vi "Merge Traces.vi"(8 "error in (no error)":errorcluster, 10 "Historical Data from Logging Database":T1, 11 "Historical Data from Archive Database":T1) -> (0 "error out":errorcluster, 3 "Merged Historical Trace":T1)   [LabVIEW 2024]
doc: "Merges the traces from the logging database and the archive database."
uses:
  Controls/Client/Historical Data.ctl
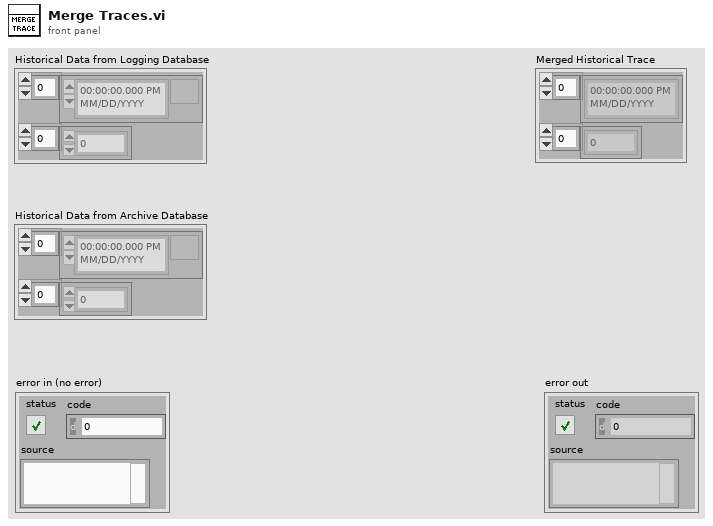
[diagram p1: front panel]
types:
  T1 = typedef "Historical Data.ctl" = cluster{"timestamps":timestamp[], "data":dbl[]}
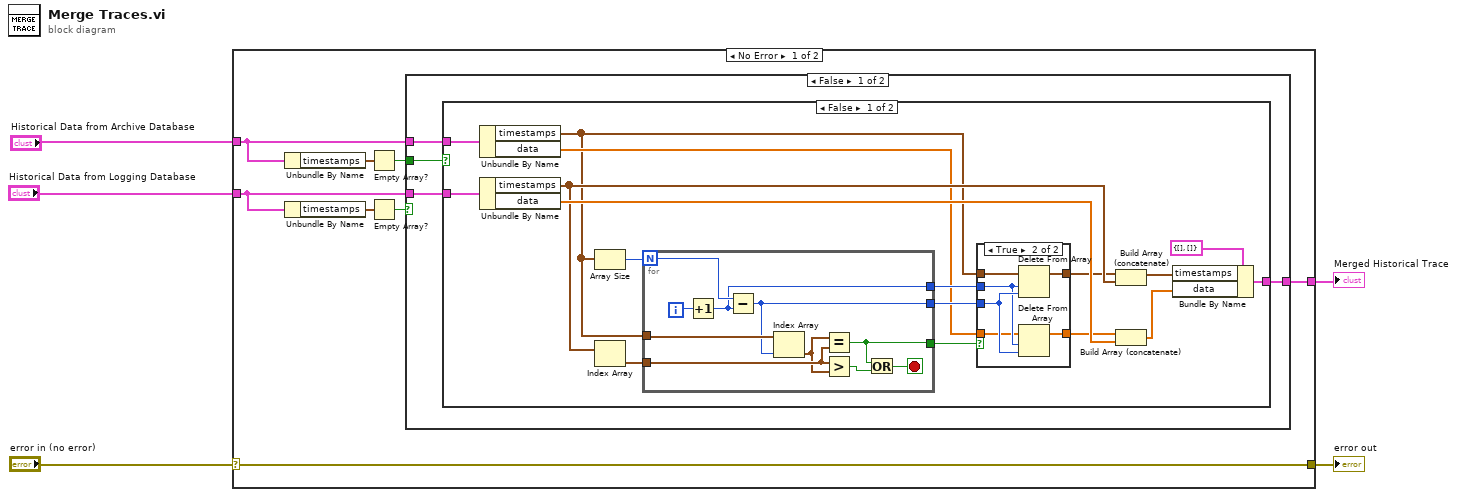
[diagram p0: block diagram]
diagram:
  n1 = case shown="No Error" "error in (no error)" {
    selector: "error in (no error)" -> [w6 w55]
    tunnel: [w6 w55] -> w4
    tunnel: "Historical Data from Archive Database" -> [w9 _]
    tunnel: "Historical Data from Logging Database" -> [w8 _]
    tunnel: [w7 _] -> w1
    frame No Error {
      n2 = Unbundle By Name(w9) -> ("timestamps"=w11:timestamp[])
      n3 = Unbundle By Name(w8) -> ("timestamps"=w13:timestamp[])
      n4 = Empty Array?(array=w11) -> (empty?=w10:bool)
      n5 = Empty Array?(array=w13) -> (empty?=w12:bool)
      n6 = case shown="False" w12 {
        tunnel: w10 -> [w17 _]
        tunnel: w8 -> [w15 w54]
        tunnel: w9 -> [w16 _]
        tunnel: [w14 w54] -> w7
        frame False {
          n7 = case shown="False" w17 {
            tunnel: w16 -> [w30 w53]
            tunnel: w15 -> [w29 _]
            tunnel: [w28 w53] -> w14
            frame False {
              n8 = Unbundle By Name(w30) -> ("timestamps"=w19:timestamp[], "data"=w22:dbl[])
              n9 = Unbundle By Name(w29) -> ("timestamps"=w26:timestamp[], "data"=w31:dbl[])
              n10 = Array Size(array=w19) -> (size(s)=w18:i32)
              n11 = Index Array(array=w26) -> (element=w27:timestamp)  [unwired: 1 in]
              n12 = for {
                N: w18 -> [w48]
                tunnel: w27 -> [w50]
                tunnel: w19 -> [w52]
                tunnel: [w46] -> w23
                tunnel: [w51] -> w25
                tunnel: [w43] -> w24
                i -> [w44]
                stop <- w47 stop-if-true
                n13 = Increment(x=w44) -> (x+1=w43:i32)
                n14 = Subtract(x=w48, y=w43) -> (x-y=w51:i32)
                n15 = Index Array(array=w52, index=w51) -> (element=w49:timestamp)
                n16 = Equal?(x=w49, y=w50) -> (x = y?=w46:bool)
                n17 = Greater?(x=w50, y=w49) -> (0:w45:bool)
                n18 = Or(x=w46, y=w45) -> (x .or. y?=w47:bool)
              }
              n19 = case shown="True" w23 {
                tunnel: w19 -> [w35 w42]
                tunnel: w25 -> [_ w40]
                tunnel: w24 -> [_ w39]
                tunnel: [w35 w41] -> w21
                tunnel: w22 -> [w36 w38]
                tunnel: [w36 w37] -> w20
                frame False {
                }
                frame True {
                  n20 = Delete From Array(array=w42, length=w39, index=w40) -> (array with subset deleted=w41:timestamp[])  [unwired: 1 out]
                  n21 = Delete From Array(array=w38, length=w39, index=w40) -> (array with subset deleted=w37:dbl[])  [unwired: 1 out]
                }
              }
              n22 = Build Array (concatenate)(w21, w26) -> (w33:timestamp[])
              n23 = Build Array (concatenate)(w20, w31) -> (w34:dbl[])
              n24 = Bundle By Name(cluster=cluster{"timestamps":timestamp[], "data":dbl[]} {"timestamps"=[], "data"=[]} ("historical trace"), "timestamps"=w33, "data"=w34) -> (w28:cluster{"timestamps":timestamp[], "data":dbl[]})
            }
            frame True {
            }
          }
        }
        frame True {
        }
      }
    }
    frame Error {
    }
  }
  "error out" <- w4
  "Merged Historical Trace" <- w1
